vi "assembly_V_SET_command.vi"(8 "error_in":errorcluster, 10 "voltage":dbl=0.001 min=0.0 max=120.0 format="%#_6f", 11 "channel":T1=enum."1") -> (0 "error_out":errorcluster, 3 "command":string)   [LabVIEW 2017]
uses:
  subVI/motech_power_supply/types/channels_enum.ctl
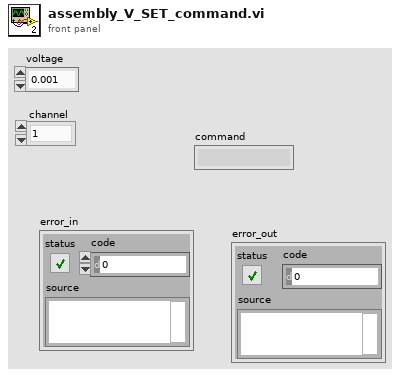
[diagram p1: front panel]
types:
  T1 = typedef "channels_enum.ctl" = enum16{"0", "1", "2"}
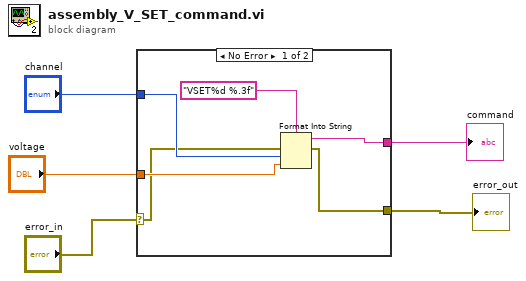
[diagram p0: block diagram]
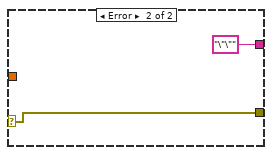
[diagram p2: hidden frame]
diagram:
  n1 = case shown="No Error" "error_in" {
    selector: "error_in" -> [w7 w12]
    tunnel: "voltage" -> [w11 _]
    tunnel: [w9 "\"\""] -> w4
    tunnel: "channel" -> [w8 _]
    tunnel: [w6 w12] -> w3
    frame No Error {
      n2 = Format Into String(format string="VSET%d %.3f", error in=w7, w8, w11) -> (resulting string=w9:string, error out=w6:errorcluster)  [unwired: 1 in]
    }
    frame Error {
    }
  }
  "command" <- w4
  "error_out" <- w3
